vi "Find all Classes in LV XML.vi"(8 "error in (no error)":errorcluster, 11 "Project Path":path) -> (0 "error out":errorcluster, 3 "Class Paths":path[](array[path]))   [LabVIEW 2020, in "Test Finder.lvclass"]
uses:
  Test Finder.lvclass
  Test Finder.lvclass/Test Finder.ctl
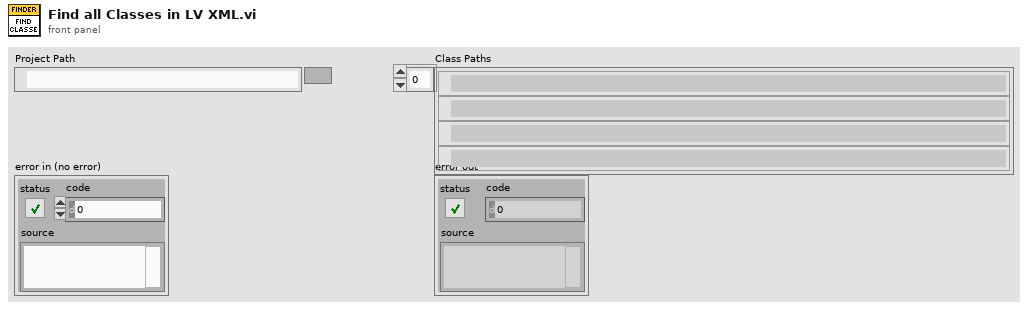
[diagram p1: front panel]
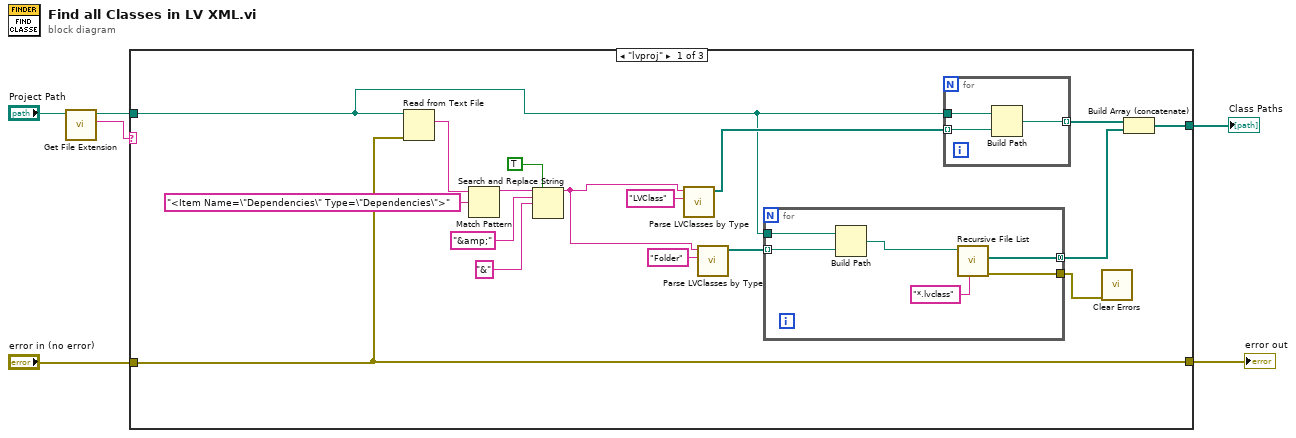
[diagram p0: block diagram]
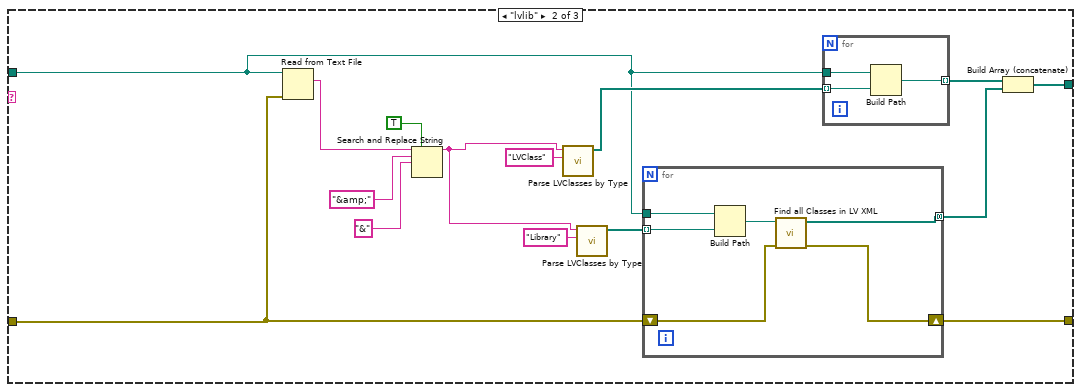
[diagram p2: hidden frame]
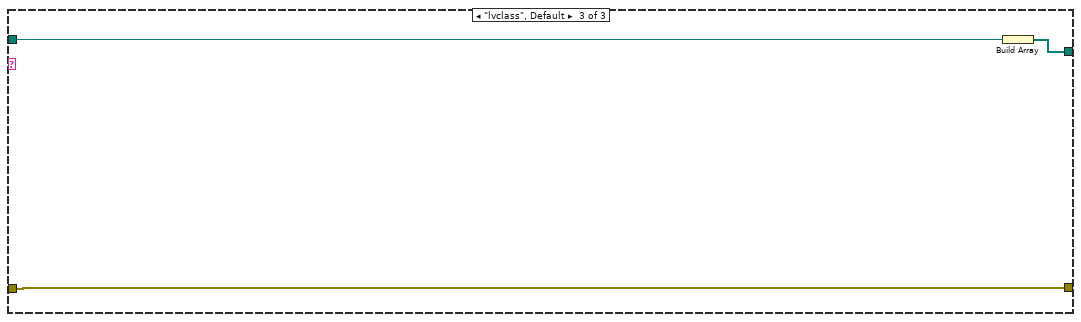
[diagram p3: hidden frame]
diagram:
  n1 = call <vilib>:"Get File Extension.vi"("file"="Project Path") -> ("lowercase file extension"=w2:string, "dup file"=w3:path)  [unwired: 6 in, 3 out]
  n2 = case shown="\"lvproj\"" w2 {
    tunnel: [w20 w44 w59] -> w6
    tunnel: "error in (no error)" -> [w8 w34 w57]
    tunnel: w3 -> [w7 w33 w58]
    tunnel: [w8 w35 w57] -> w1
    frame "lvproj" {
      n3 = Read from Text File(file (use dialog)=w7, error in=w8) -> (text=w14:string)  [unwired: 2 in, 3 out]
      n4 = Match Pattern(string=w14, regular expression="<Item Name=\"Dependencies\" Type=\"Dependencies\">") -> (before substring=w13:string)  [unwired: 1 in, 3 out]
      n5 = Search and Replace String(replace all?=TRUE ("replace all? (F)"), input string=w13, search string="&amp;", replace string="&" ("search string")) -> (result string=w12:string)  [unwired: 4 in, 3 out]
      n6 = call "Parse LVClasses by Type.vi"("Type"="LVClass", "Input"=w12) -> ("Relative Paths"=w23:path[])  [unwired: 9 in]
      n7 = call "Parse LVClasses by Type.vi"("Type"="Folder", "Input"=w12) -> ("Relative Paths"=w18:path[])  [unwired: 9 in]
      n8 = for {
        tunnel: w18 -> [w27] mode=indexing
        tunnel: [w31] -> w17 mode=concatenating
        tunnel: [w30] -> w16
        tunnel: w7 -> [w29]
        n9 = Build Path(base path=w29, name or relative path=w27) -> (appended path=w28:path)
        n10 = call <vilib>:"Recursive File List.vi"("pattern"="*.lvclass", "Folder Path"=w28) -> ("error out"=w30:errorcluster, "All Files in Dir"=w31:path[])  [unwired: 5 in, 3 out]
      }
      n11 = for {
        tunnel: w7 -> [w26]
        tunnel: w23 -> [w25] mode=indexing
        tunnel: [w24] -> w22 mode=indexing
        n12 = Build Path(base path=w26, name or relative path=w25) -> (appended path=w24:path)
      }
      n13 = call <vilib>:"Clear Errors.vi"("error in (no error)"=w16) -> ()  [unwired: 5 in, 2 out]
      n14 = Build Array (concatenate)(w22, w17) -> (w20:path[])
    }
    frame "lvlib" {
      n15 = Read from Text File(file (use dialog)=w33, error in=w34) -> (text=w40:string)  [unwired: 2 in, 3 out]
      n16 = Search and Replace String(replace all?=TRUE ("replace all? (F)"), input string=w40, search string="&amp;", replace string="&" ("search string")) -> (result string=w39:string)  [unwired: 4 in, 3 out]
      n17 = call "Parse LVClasses by Type.vi"("Type"="LVClass", "Input"=w39) -> ("Relative Paths"=w47:path[])  [unwired: 9 in]
      n18 = call "Parse LVClasses by Type.vi"("Type"="Library", "Input"=w39) -> ("Relative Paths"=w42:path[])  [unwired: 9 in]
      n19 = for {
        tunnel: w42 -> [w55] mode=indexing
        tunnel: [w53] -> w41 mode=concatenating
        tunnel: w33 -> [w56]
        shift-right: [w51] -> w35
        shift-left: w34 -> [w52]
        n20 = Build Path(base path=w56, name or relative path=w55) -> (appended path=w54:path)
        n21 = call "Find all Classes in LV XML.vi"("error in (no error)"=w52, "Project Path"=w54) -> ("error out"=w51:errorcluster, "Class Paths"=w53:path[])  [unwired: 8 in]
      }
      n22 = for {
        tunnel: w33 -> [w50]
        tunnel: w47 -> [w49] mode=indexing
        tunnel: [w48] -> w46 mode=indexing
        n23 = Build Path(base path=w50, name or relative path=w49) -> (appended path=w48:path)
      }
      n24 = Build Array (concatenate)(w46, w41) -> (w44:path[])
    }
    frame "lvclass", Default {
      n25 = Build Array(w58) -> (w59:path[])
    }
  }
  "error out" <- w1
  "Class Paths" <- w6
